vi "LINC Daemon Manager.vi"(5 "target name":string, 7 "mode":T1, 8 "error in (no error)":errorcluster) -> (0 "error out":errorcluster, 2 "running":bool)   [LabVIEW 2018, in "STEPkgDriver_LINC.lvlib"]
uses:
  STEPkgDriver_LINC.lvlib
  LINC Daemon Manager Mode.ctl
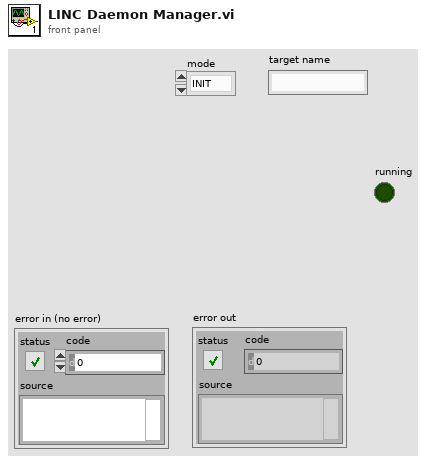
[diagram p1: front panel]
types:
  T1 = typedef "STEPkgDriver_LINC.lvlib/LINC Daemon Manager Mode.ctl" = enum16{"INIT", "CLEAR", "GET"}
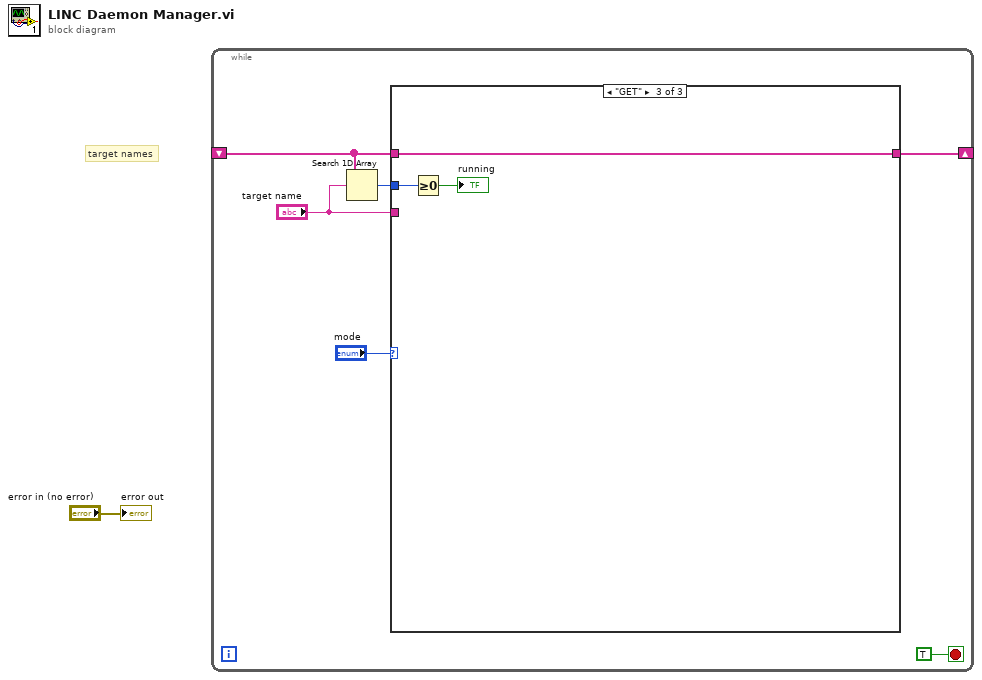
[diagram p0: block diagram]
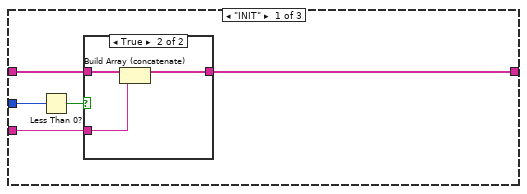
[diagram p2: hidden frame]
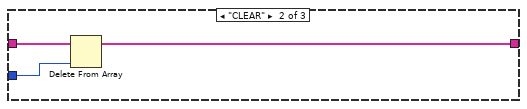
[diagram p4: hidden frame]
diagram:
  # "target names"
  n1 = while {
    shift-right: [w5] -> _
    shift-left: _ -> [w4]
    stop <- TRUE stop-if-true
    n2 = Search 1D Array(1D array=w4, element="target name") -> (index of element=w2:i32)  [unwired: 1 in]
    n3 = case shown="\"GET\"" "mode" {
      tunnel: "target name" -> [w12 _ _]
      tunnel: w4 -> [w11 w19 w22]
      tunnel: [w10 w18 w22] -> w5
      tunnel: w2 -> [w9 w17 w21]
      frame "INIT" {
        n4 = Less Than 0?(x=w9) -> (x < 0?=w8:bool)
        n5 = case shown="True" w8 {
          tunnel: w12 -> [_ w16]
          tunnel: w11 -> [w13 w15]
          tunnel: [w13 w14] -> w10
          frame False {
          }
          frame True {
            n6 = Build Array (concatenate)(w15, w16) -> (w14:string[])
          }
        }
      }
      frame "CLEAR" {
        n7 = Delete From Array(array=w19, index=w17) -> (array with subset deleted=w18:string[])  [unwired: 1 in, 1 out]
      }
      frame "GET" {
        n8 = Greater Or Equal To 0?(x=w21) -> (x >= 0?=→"running":bool)
      }
    }
  }
  "error out" <- "error in (no error)"
